vi "Laser-Set-Energy.vi"(2 "error in (no error)":errorcluster, 3 "SetLaserEnergy":dbl=0.8, 4 "VISA resource name":refnum<visa-resource-name>) -> (0 "error out":errorcluster, 1 "VISA resource name out":refnum<visa-resource-name>)   [LabVIEW 2013]
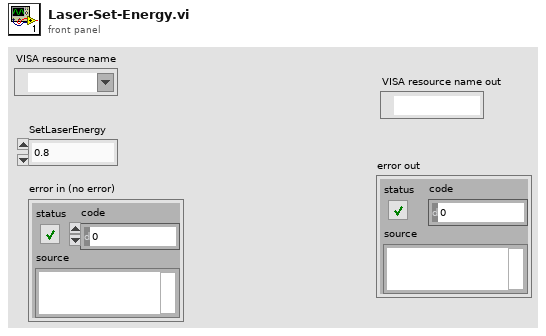
[diagram p1: front panel]
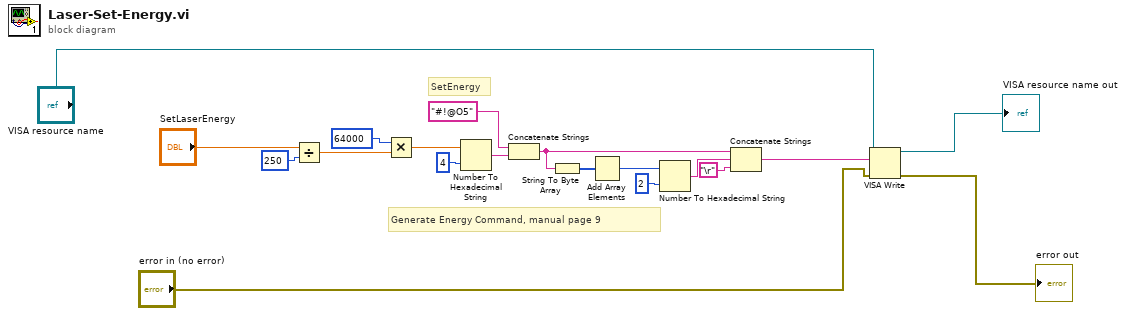
[diagram p0: block diagram]
diagram:
  # "Generate Energy Command, manual page 9"
  # "SetEnergy"
  n1 = Divide(x="SetLaserEnergy", y=250) -> (x/y=w9:dbl)
  n2 = Multiply(x=64000, y=w9) -> (x*y=w7:dbl)
  n3 = Number To Hexadecimal String(1:i16 4 ("width (-)"), 2:w7) -> (0:w18:string)
  n4 = Concatenate Strings("#!@O5" ("string"), w18) -> (w14:string)
  n5 = String To Byte Array(string=w14) -> (unsigned byte array=w17:u8[])
  n6 = Add Array Elements(numeric array=w17) -> (sum=w16:u8)
  n7 = Number To Hexadecimal String(1:i16 2 ("width (-)"), 2:w16) -> (0:w13:string)
  n8 = Concatenate Strings(w14, w13, "\r") -> (w5:string)
  n9 = VISA Write(VISA resource name="VISA resource name", write buffer=w5, error in (no error)="error in (no error)") -> (VISA resource name out=→"VISA resource name out":refnum<visa-resource-name>, error out=→"error out":errorcluster)  [unwired: 1 out]
